vi "fitting is almost done song.vi"   [LabVIEW 2016]
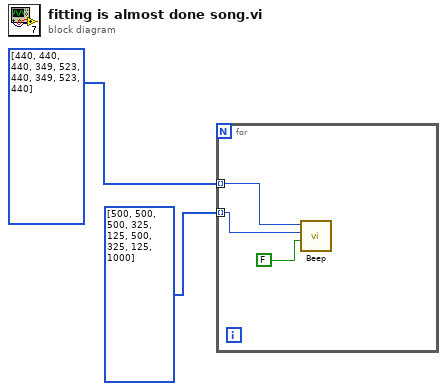
[diagram p0: block diagram]
diagram:
  n1 = for {
    tunnel: i32[] [500, 500, 500, 325, 125, 500, 325, 125, 1000] -> [w4] mode=indexing
    tunnel: i32[] [440, 440, 440, 349, 523, 440, 349, 523, 440] -> [w3] mode=indexing
    n2 = call <vilib>:"Beep.vi"("use system alert? (T)"=FALSE, "duration (msec)"=w4, "frequency (Hz)"=w3) -> ()  [unwired: 9 in]
  }
